vi "Exemplo.vi"() -> ()   [LabVIEW 2015]
uses:
  <vilib>/NXT/Subs/LVHSConnector.ctl
  <vilib>/NXT/LegoClasses/BrickReference/BrickReference.lvclass
  <vilib>/NXT/Subs/MotorOutput.ctl
  <vilib>/NXT/Block Support/NXT_InputPort.ctl
  <vilib>/NXT/Block Support/NXT_ButtonSelector.ctl
  <vilib>/NXT/Dual Mode Library/Display/clearDisplay.vi
  <vilib>/NXT/Dual Mode Library/Sensors/readNXTButton.vi
panel:
  out "DESV":bool
  out "STOP":bool
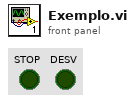
[diagram p1: front panel]
types:
  T1 = typedef "MotorOutput.ctl" = u8
  T2 = typedef "LVHSConnector.ctl" = refnum<class "BrickReference.lvclass">
  T3 = typedef "NXT_InputPort.ctl" = u32
  T4 = typedef "NXT_ButtonSelector.ctl" = u16
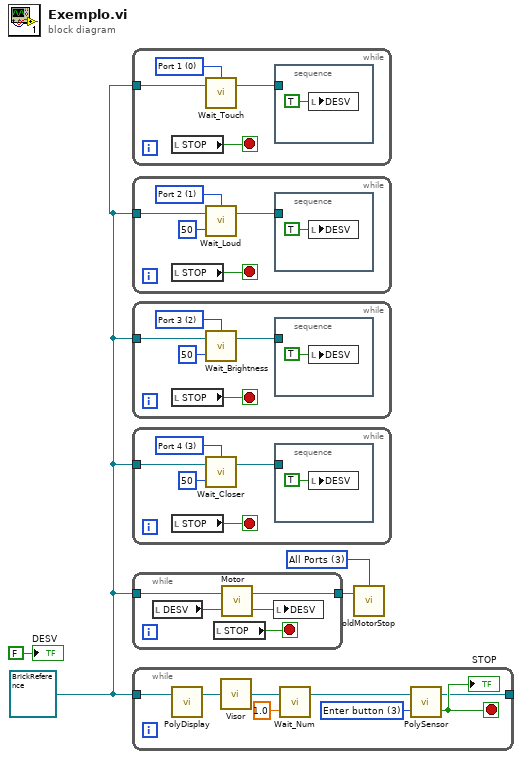
[diagram p0: block diagram]
diagram:
  w2 = T1 3 items=["Port A"=0, "Port B"=1, "Port C"=2, "Ports A & B"=4, "Ports A & C"=5, "Ports B & C"=6, "All Ports"=3] ("Output Port (All Ports)")
  w1 = T2 refnum ("NXT/EV3")
  n1 = while {
    tunnel: w1 -> [w7]
    stop <- w8 stop-if-true
    w6 = T3 0 items=["Port 1", "Port 2", "Port 3", "Port 4"] ("Port (Port 1)")
    n2 = local read "STOP"() -> (w8:bool)
    n3 = call <vilib>:"Wait_Touch.vi"("NXT/EV3"=w7, "Port (Port 1)"=w6) -> ("NXT/EV3"=w5:T2)  [unwired: 2 in]
    n4 = stacked-sequence {
      tunnel: w5 -> [_]
      frame #0 {
        n5 = local write "DESV"(TRUE ("DESV")) -> ()
      }
    }
  }
  n6 = while {
    tunnel: w1 -> [w13]
    stop <- w14 stop-if-true
    w12 = T3 1 items=["Port 1", "Port 2", "Port 3", "Port 4"] ("Port (Port 1)")
    n7 = local read "STOP"() -> (w14:bool)
    n8 = call <vilib>:"Wait_Loud.vi"("Loudness (40)"=u8 50, "NXT/EV3"=w13, "Port (Port 2)"=w12) -> ("NXT/EV3"=w11:T2)  [unwired: 1 in]
    n9 = stacked-sequence {
      tunnel: w11 -> [_]
      frame #0 {
        n10 = local write "DESV"(TRUE ("DESV")) -> ()
      }
    }
  }
  n11 = while {
    tunnel: w1 -> [w19]
    stop <- w20 stop-if-true
    w18 = T3 2 items=["Port 1", "Port 2", "Port 3", "Port 4"] ("Port (Port 1)")
    n12 = local read "STOP"() -> (w20:bool)
    n13 = call <vilib>:"Wait_Brightness.vi"("Brightness (40)"=i16 50, "NXT/EV3"=w19, "Port (Port 3)"=w18) -> ("NXT/EV3"=w17:T2)  [unwired: 1 in]
    n14 = stacked-sequence {
      tunnel: w17 -> [_]
      frame #0 {
        n15 = local write "DESV"(TRUE ("DESV")) -> ()
      }
    }
  }
  n16 = while {
    tunnel: w1 -> [w25]
    stop <- w26 stop-if-true
    w24 = T3 3 items=["Port 1", "Port 2", "Port 3", "Port 4"] ("Port (Port 1)")
    n17 = local read "STOP"() -> (w26:bool)
    n18 = call <vilib>:"Wait_Closer.vi"("Distance (40)"=i16 50, "NXT/EV3"=w25, "Port (Port 4)"=w24) -> ("NXT/EV3"=w23:T2)  [unwired: 1 in]
    n19 = stacked-sequence {
      tunnel: w23 -> [_]
      frame #0 {
        n20 = local write "DESV"(TRUE ("DESV")) -> ()
      }
    }
  }
  n21 = while {
    tunnel: w1 -> [w30]
    tunnel: [w28] -> w3
    stop <- w32 stop-if-true
    n22 = local read "DESV"() -> (w31:bool)
    n23 = local read "STOP"() -> (w32:bool)
    n24 = call "Motor.vi"("DESV-IN"=w31, "BrickReference in"=w30) -> ("DESV-OUT"=w29:bool, "BrickReference out"=w28:T2)
    n25 = local write "DESV"(w29) -> ()
  }
  n26 = while {
    tunnel: w1 -> [w38]
    tunnel: [w33] -> _
    stop <- w39 stop-if-true
    w40 = T4 3 items=["Enter button"=3, "Left button"=2, "Right button"=1, "Up Button"=4, "Down Button"=5] ("Button (Enter button)")
    n27 = call-poly <vilib>:"PolyDisplay.vi"("NXT/EV3"=w38) -> ("NXT/EV3"=w37:T2)  [unwired: 3 in]
    n28 = call "Visor.vi"("Line IN"=w37) -> ("Line OUT"=w36:T2)
    n29 = call <vilib>:"Wait_Num.vi"("Time (1 sec)"=sgl 1.0, "NXT/EV3"=w36) -> ("NXT/EV3"=w35:T2)  [unwired: 2 in]
    n30 = call-poly <vilib>:"PolySensor.vi"("Button (Enter button)"=w40, "NXT/EV3"=w35) -> ("Yes/No"=w39:bool, "NXT/EV3"=w33:T2)  [unwired: 1 in]
    "STOP" <- w39
  }
  n31 = call <vilib>:"oldMotorStop.vi"("NXT/EV3"=w3, "Output Port (All Ports)"=w2) -> ()  [unwired: 2 in, 1 out]
  "DESV" <- FALSE ("MOVE")
